vi "Read Array of Sequences.vi"(8 "error in (no error)":errorcluster, 11 "Scheduler in":refnum<class "Scheduler.lvclass">) -> (0 "error out":errorcluster, 2 "Array of Seqs":refnum<class "Sequence of SBlocks.lvclass">[](array[class]), 3 "Scheduler out":refnum<class "Scheduler.lvclass">)   [LabVIEW 2020, in "Scheduler.lvlib" / "Scheduler.lvclass"]
uses:
  Scheduler.lvclass
  Run Utilities/Sequence of SBlocks/Sequence of SBlocks.lvclass
  Scheduler.lvclass/Scheduler.ctl
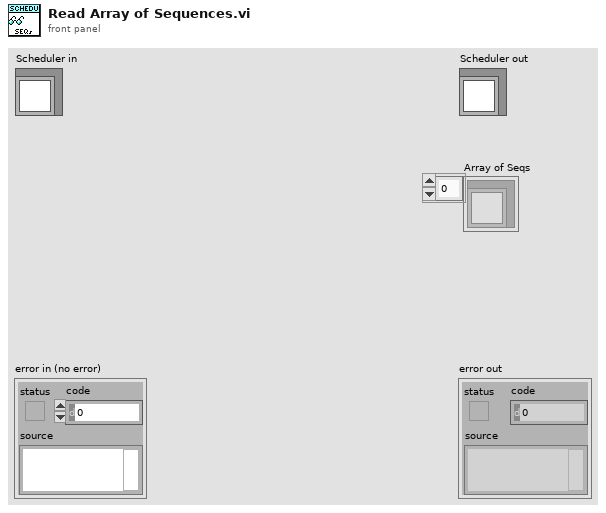
[diagram p1: front panel]
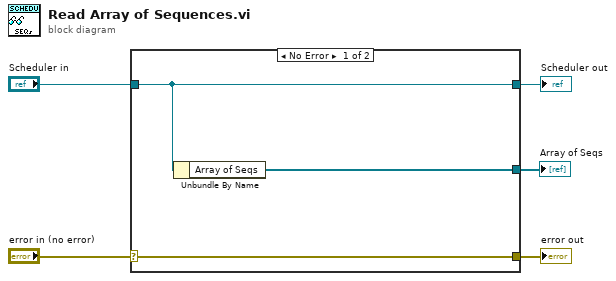
[diagram p0: block diagram]
diagram:
  n1 = case shown="No Error" "error in (no error)" {
    selector: "error in (no error)" -> [w8 w9]
    tunnel: [w8 w9] -> w4
    tunnel: [w7 w10] -> w2
    tunnel: "Scheduler in" -> [w7 w10]
    tunnel: [w6 _] -> w1
    frame No Error {
      n2 = Unbundle By Name(w7) -> ("Array of Seqs"=w6:refnum<class "Sequence of SBlocks.lvclass">[])
    }
    frame Error {
    }
  }
  "error out" <- w4
  "Scheduler out" <- w2
  "Array of Seqs" <- w1
